vi "글로벌변수_1.vi"() -> ()   [LabVIEW 2013]
panel:
  in  "정지":bool
  out "웨이브폼 차트":dbl(graph)
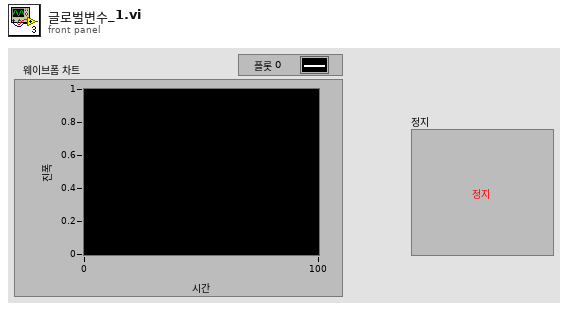
[diagram p1: front panel]
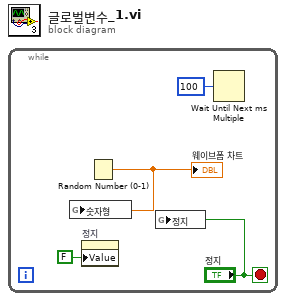
[diagram p0: block diagram]
diagram:
  n1 = while {
    stop <- "정지" stop-if-true
    n2 = property on="정지" class="Bool (엄격한)"("Value"=FALSE ("정지")) -> ()  [unwired: 2 in, 2 out]
    n3 = Random Number (0-1)() -> (number: 0 to 1=w3:dbl)
    "웨이브폼 차트" <- w3
    n4 = global write "글로벌_변수VI.vi" "숫자형"(w3) -> ()
    n5 = global write "글로벌_변수VI.vi" "정지"("정지") -> ()
    n6 = Wait Until Next ms Multiple(millisecond multiple=u32 100 ("ms 배수")) -> ()  [unwired: 1 out]
  }
